vi "Delacor_lib_QMH_Property Node (DQMH Error Debug).vi"   [LabVIEW 2023]
doc: "____\nDQMH Framework: Palette 7.1.0.1503\nCopyright (c) 2025, DQMH Consortium"
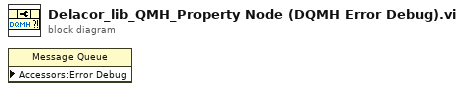
[diagram p0: block diagram]
diagram:
  n1 = property class="Message Queue" props=["Accessors:Error Debug"]() -> ()  [unwired: 3 in, 2 out]
